vi "DcPreBootTest.vi"(0 "String in":refnum<vi>, 1 "lsl/hsl limit":dbl[](array[numeric]) format="%#_13g", 5 "reference in":refnum<vi>, 9 "concatenated string":string, 11 "error in (no error)":errorcluster, 12 "seconds to wait":dbl format="%#_13g") -> (3 "DcLow?(t= low)":bool, 6 "concatenated stringout":string, 14 "FlagDC?(t)":bool, 15 "error out":errorcluster)   [LabVIEW 2018]
uses:
  Initialize References/Station References Global.vi
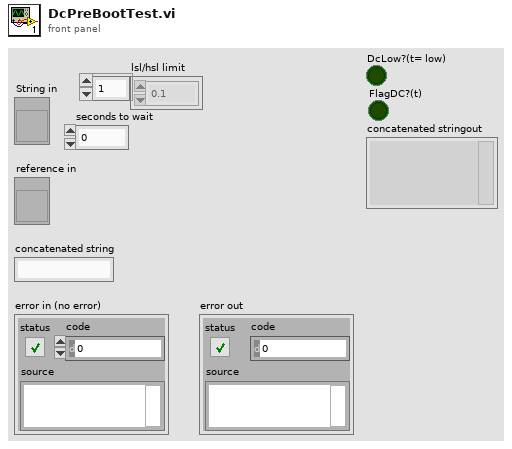
[diagram p1: front panel]
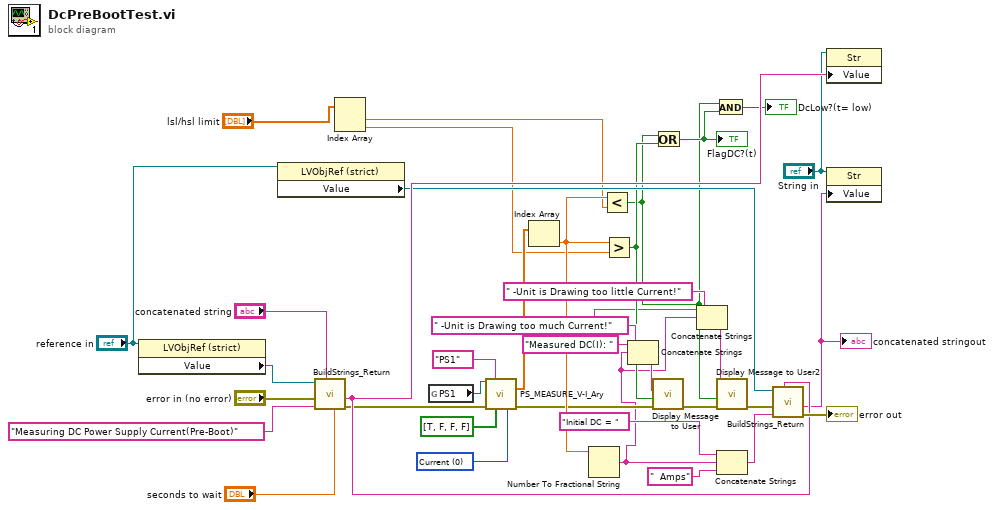
[diagram p0: block diagram]
diagram:
  w4 = "Measured DC(I): " ("string")
  w24 = 0 items=["Current", "Voltage"] ("Measurement Type (1: Voltage)")
  n1 = property class="LVObjRef (strict)"(reference="reference in") -> ("Value"=w27:refnum<vi>)  [unwired: 1 in, 2 out]
  n2 = property class="LVObjRef (strict)"(reference="reference in") -> ("Value"=w29:refnum<vi>)  [unwired: 1 in, 2 out]
  n3 = call "BuildStrings_Return.vi"("seconds to wait"="seconds to wait", "Input String"="concatenated string", "New String"="Measuring DC Power Supply Current(Pre-Boot)", "error in (no error)"="error in (no error)", "reference"=w27) -> ("error out"=w18:errorcluster, "concatenated string"=w30:string)  [unwired: 4 in, 1 out]
  n4 = Index Array(array="lsl/hsl limit") -> (element #1=w7:dbl, element #2=w2:dbl)  [unwired: 2 in]
  n5 = global read "Station References Global.vi" "PS1"() -> (w19:refnum<visa-resource-name>)
  n6 = call "PS_MEASURE_V-I_Ary.vi"("VISA resource name"=w19, "SEL_PS"="PS1", "error in (no error)"=w18, "Array 2"=bool[] [TRUE, FALSE, FALSE, FALSE], "Measurement Type (1: Voltage)"=w24) -> ("Array"=w17:dbl[], "error out"=w20:errorcluster)  [unwired: 8 in, 1 out]
  n7 = Index Array(array=w17) -> (element=w35:dbl)  [unwired: 1 in]
  n8 = Number To Fractional String(number=w35) -> (F-format string=w3:string)  [unwired: 3 in]
  n9 = Less?(x=w35, y=w7) -> (x < y?=w11:bool)
  n10 = Greater?(x=w35, y=w2) -> (0:w13:bool)
  n11 = Concatenate Strings(w4, w3, " -Unit is Drawing too much Current!" ("initial string")) -> (w5:string)
  n12 = call "Display Message to User"("error in (no error)"=w20, "Enable"=w13, "Message"=w5) -> ("error out"=w16:errorcluster)  [unwired: 7 in, 1 out]
  n13 = Or(x=w11, y=w13) -> (x .or. y?=w12:bool)
  "FlagDC?(t)" <- w12
  n14 = Concatenate Strings(w4, w3, " -Unit is Drawing too little Current!" ("initial string")) -> (w6:string)
  n15 = And(x=w11, y=w12) -> (x .and. y?=→"DcLow?(t= low)":bool)
  n16 = call "Display Message to User2"("error in (no error)"=w16, "Enable"=w11, "Message"=w6) -> ("error out"=w28:errorcluster)  [unwired: 7 in, 1 out]
  n17 = Concatenate Strings("Initial DC = " ("New String"), w3, "  Amps" ("string")) -> (w34:string)
  n18 = call "BuildStrings_Return.vi"("Input String"=w30, "New String"=w34, "error in (no error)"=w28, "reference"=w29) -> ("error out"=→"error out":errorcluster, "concatenated string"=w9:string)  [unwired: 5 in, 1 out]
  "concatenated stringout" <- w9
  n19 = property class="Str"(reference="String in", "Value"=w30) -> ()  [unwired: 1 in, 2 out]
  n20 = property class="Str"(reference="String in", "Value"=w9) -> ()  [unwired: 1 in, 2 out]
